vi "WriteGpio.vi"(8 "error in (no error)":errorcluster, 9 "GPIO #2 in":u32, 10 "GPIO #1 in":u32, 11 "FpgaInterface in":refnum<class "FpgaInterface.lvclass">) -> (0 "error out":errorcluster, 3 "FpgaInterface out":refnum<class "FpgaInterface.lvclass">)   [LabVIEW 2017, in "FpgaInterface.lvclass"]
uses:
  FpgaInterface.lvclass
  FpgaInterface.lvclass/FpgaInterface.ctl
  <vilib>/Utility/error.llb/Error Cluster From Error Code.vi
  <vilib>/rvi/errors/niLvFpgaAdjustHostInterfaceError.vi
  <vilib>/rvi/interface/nirviReadWriteControl/nirviReadWriteControl.xnode
  NiFpgaLv.dll
  <vilib>/rvi/interface/Simulation/niFpgaSimulationCallBeginRW.vi
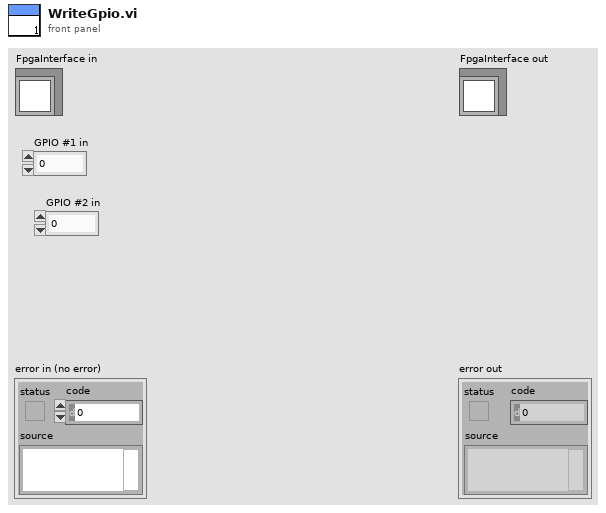
[diagram p1: front panel]
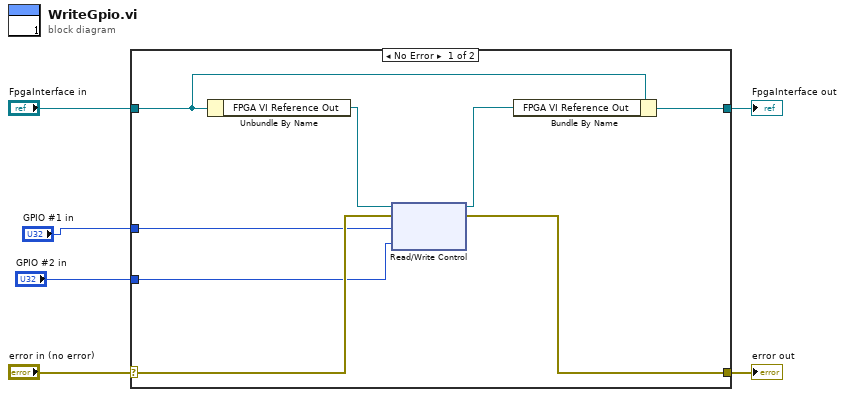
[diagram p0: block diagram]
diagram:
  n1 = case shown="No Error" "error in (no error)" {
    selector: "error in (no error)" -> [w13 w16]
    tunnel: [w12 w16] -> w5
    tunnel: [w7 w15] -> w3
    tunnel: "FpgaInterface in" -> [w8 w15]
    tunnel: "GPIO #1 in" -> [w11 _]
    tunnel: "GPIO #2 in" -> [w10 _]
    frame No Error {
      n2 = Unbundle By Name(w8) -> ("FPGA VI Reference Out"=w14:refnum<k20>)
      n3 = xnode "Read/Write Control"("FPGA VI Reference In"=w14, "error in"=w13, "GPIO #1 in"=w11, "GPIO #2 in"=w10) -> ("FPGA VI Reference Out"=w9:refnum<k20>, "error out"=w12:errorcluster)
      n4 = Bundle By Name(cluster=w8, "FPGA VI Reference Out"=w9) -> (w7:refnum<class "FpgaInterface.lvclass">)
    }
    frame Error {
    }
  }
  "error out" <- w5
  "FpgaInterface out" <- w3
